vi "Create Tx Sequence.vi"(0 "# Guard Bits (2)":i32=2, 1 "Block Length (-1)":i32=-1, 2 "PN sequence order (9)":i32=9, 5 "# Sync Bits (20)":i32=20, 7 "Reset? (T)":bool=TRUE, 9 "Send Preamble on reset? (T)":bool=TRUE, 11 "error in (no error)":errorcluster, 12 "# Message Bits":i32=1000, 13 "seed for message":i32=-692093454 format="%.0x") -> (4 "Output Bit Stream":i8[](array[numeric]), 6 "Last Sync Pattern":i8[](array[numeric]), 8 "Last Guard Pattern":i8[](array[numeric]), 15 "error out":errorcluster)   [LabVIEW 2019]
uses:
  <vilib>/addons/Modulation/Digital/General/MT Generate Bits (Galois, PN Order).vi
  <vilib>/addons/Modulation/Digital/Support/Common/Validators/mod_Generate Bits Validate.vi
  <vilib>/addons/Modulation/Analog/support/mod_Set Error Source.vi
  <vilib>/addons/Modulation/Digital/General/subVIs/mod_Generate Bits PN Sequence.vi
  <vilib>/addons/Modulation/Digital/General/MT Generate Bits (User Defined).vi
  <vilib>/addons/Modulation/niDMT.lvlib
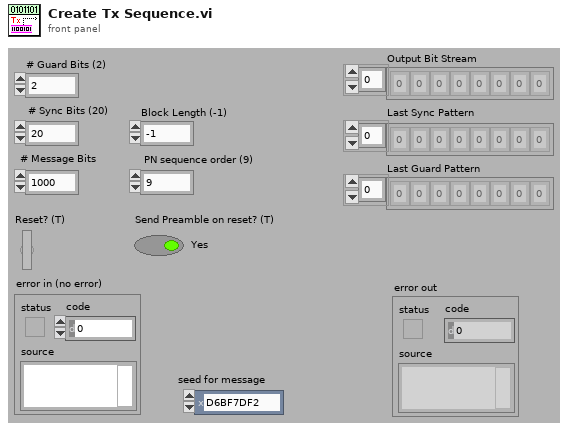
[diagram p1: front panel]
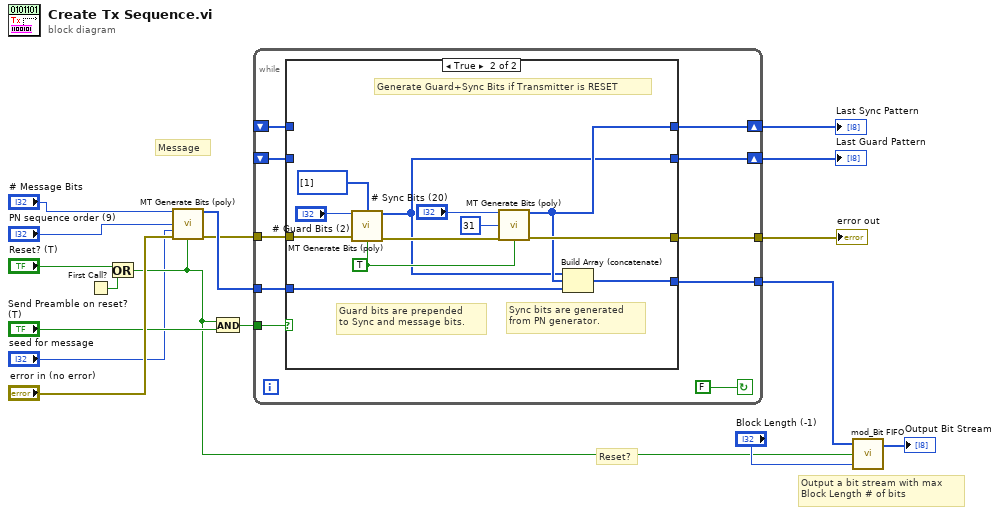
[diagram p0: block diagram]
diagram:
  # "Output a bit stream with max\nBlock Length # of bits"
  # "Reset?"
  # "Message"
  n1 = First Call?() -> (First Call?: T/F=w13:bool)
  n2 = Or(x="Reset? (T)", y=w13) -> (x .or. y?=w2:bool)
  n3 = call-poly <vilib>:"MT Generate Bits (poly).vi"("total bits (128)"="# Message Bits", "PN sequence order (9)"="PN sequence order (9)", "seed in (0xD6BF7DF2)"="seed for message", "error in (no error)"="error in (no error)", "reset? (T)"=w2) -> ("output bit stream"=w16:i8[], "error out"=w10:errorcluster)  [unwired: 9 out]
  n4 = And(x=w2, y="Send Preamble on reset? (T)") -> (x .and. y?=w12:bool)
  n5 = while {
    tunnel: w16 -> [w27]
    tunnel: w12 -> [w26]
    tunnel: w10 -> [w25]
    tunnel: [w24] -> w9
    tunnel: [w23] -> w8
    shift-right: [w21] -> w5
    shift-left: _ -> [w20]
    shift-right: [w19] -> w3
    shift-left: _ -> [w18]
    stop <- FALSE continue-if-true
    n6 = case shown="True" w26 {
      tunnel: w27 -> [w31 w43]
      tunnel: [w31 w42] -> w23
      tunnel: w25 -> [w30 w35]
      tunnel: [w30 w41] -> w24
      tunnel: [w29 w39] -> w21
      tunnel: w20 -> [w29 _]
      tunnel: [w28 w34] -> w19
      tunnel: w18 -> [w28 _]
      frame False {
        # "Only generate the message bits since RESET=False."
      }
      frame True {
        w37 = TRUE ("Reset? (T)")
        # "Generate Guard+Sync Bits if Transmitter is RESET"
        # "Guard bits are prepended\nto Sync and message bits."
        # "Sync bits are generated \nfrom PN generator."
        n7 = call-poly <vilib>:"MT Generate Bits (poly).vi"("total bits (128)"="# Guard Bits (2)", "user base bit pattern"=i8[] [1], "error in (no error)"=w35, "reset? (T)"=w37) -> ("output bit stream"=w34:i8[], "error out"=w38:errorcluster)  [unwired: 10 out]
        n8 = call-poly <vilib>:"MT Generate Bits (poly).vi"("total bits (128)"="# Sync Bits (20)", "PN sequence order (9)"=31, "error in (no error)"=w38, "reset? (T)"=w37) -> ("output bit stream"=w39:i8[], "error out"=w41:errorcluster)  [unwired: 1 in, 9 out]
        n9 = Build Array (concatenate)(w34, w39, w43) -> (w42:i8[])
      }
    }
  }
  "error out" <- w9
  "Last Sync Pattern" <- w5
  "Last Guard Pattern" <- w3
  n10 = call <vilib>:"mod_Bit FIFO.vi"("Block Length (-1 output all)"="Block Length (-1)", "Reset?"=w2, "Input Bit Stream"=w8) -> ("Output Bit Stream"=→"Output Bit Stream":i8[])  [unwired: 1 out]
